vi "GetFPGAStatus.vi"(0 "FPGA in":refnum<queue>) -> (4 "FPGA out":refnum<queue>, 6 "Connected":bool, 8 "Acquiring":bool, 10 "Discrete Sweep":bool, 14 "Parameters Ok":bool, 15 "Demodulation":bool)   [LabVIEW 2019, in "FPGA.lvlib"]
uses:
  FPGA.lvlib
  FPGA.ctl
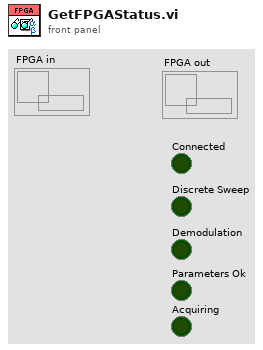
[diagram p1: front panel]
types:
  T1 = typedef "FPGA.lvlib/FPGA.ctl" = cluster{"Start freq. [Hz]":dbl, "Sweep duration [s]":dbl, "Freq. step [Hz]":dbl, "DAC Sample Rate":dbl, "ADC Sample Rate":dbl, "CMD port":u16, "DFAST port":u16, "CMD ID":refnum<k16>, "DFAST ID":refnum<k16>, "CMD error out":errorcluster, "FPGA IP":string, "DFAST error out ":errorcluster, "Stop freq. [Hz]":dbl, "Discrete sweep":bool, "Initial NCO":u32, "Difference NCO":i32, "step NCO":i64, "Final NCO":u32, "clocks for step":u32, "demodulation":bool, "NCO Phase Precision":u32, "NCO Sample Rate":dbl, "Time for step [s]":dbl, "NCO freq. resolution":dbl, "Sweep speed [Hz/s]":dbl, "Connected":bool, "Slew Rate [V/us]":dbl, "Parameters_ok":bool, "Amplitude [mVpp]":dbl, "Scale Factor":fxp<+,16,0>, "Acquiring":bool, "DAC-ADC Latency":u16, "Digital Gain":i32, "Number of steps":i32, "Averaging preferred":bool, "Filter Order":u32, "Settling":enum16{"99%", "99,9%"}}
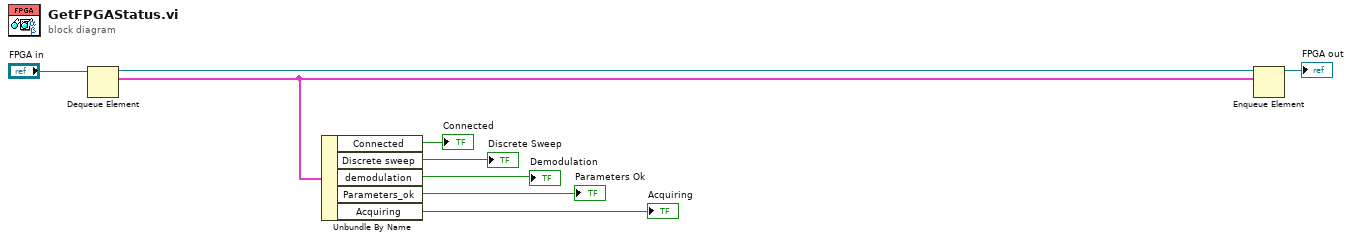
[diagram p0: block diagram]
diagram:
  n1 = Dequeue Element(queue="FPGA in") -> (queue out=w7:refnum<queue>, element=w6:T1)  [unwired: 2 in, 2 out]
  n2 = Unbundle By Name(w6) -> ("Connected"=→"Connected":bool, "Discrete sweep"=→"Discrete Sweep":bool, "demodulation"=→"Demodulation":bool, "Parameters_ok"=→"Parameters Ok":bool, "Acquiring"=→"Acquiring":bool)
  n3 = Enqueue Element(queue=w7, element=w6) -> (queue out=→"FPGA out":refnum<queue>)  [unwired: 2 in, 2 out]
